vi "边沿.vi"(10 "IN":bool) -> (0 "下降沿":bool, 3 "上升沿":bool)   [LabVIEW 2014]
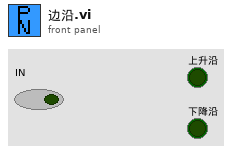
[diagram p1: front panel]
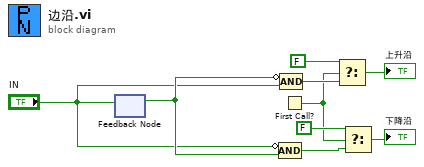
[diagram p0: block diagram]
diagram:
  n1 = feedback #1() -> (w9:bool)  [unwired: 1 in]
  n2 = feedback-in #1("IN") -> ()
  n3 = Compound Arithmetic op=AND(invert "IN", w9) -> (w4:bool)
  n4 = Compound Arithmetic op=AND(invert w9, "IN") -> (w7:bool)
  n5 = First Call?() -> (First Call?: T/F=w3:bool)
  n6 = Select(t=FALSE, s=w3, f=w7) -> (s? t:f=→"上升沿":bool)
  n7 = Select(t=FALSE, s=w3, f=w4) -> (s? t:f=→"下降沿":bool)
